vi "MS SQL_Read_TS_Routing.vi"(5 "Pokeyoke?":bool, 6 "PKYK Ref":refnum<vi>[](array[refnum]), 8 "error in (no error)":errorcluster, 11 "Ref in":T2={"MS SQL Connection"=refnum, "UDL File"=path "", "Time"="", "DCODE"="", "WIP+1"=0, "MC No?"=0, "POKAYOKE?"=FALSE, "Expected Result"="", "Result [Status]"="", "Clock"=0.0, "RFID"="", "WIP Queue"=refnum, "TS Parameter"={"ProfitCenterCode"="", "LineCode"="", "WorkOrderNumber"="", "Model"="", "Model_with_Prefix"="", "VendorCode"="", "SetParameterDateCode"="", "PokaYoke"=0, "Target"=1, "Live_DateCode"="", "CustomerPartNumber"="", "Hand"="", "sBarcode"=FALSE, "FCA"=0, "Ent_Stamp"=timestamp(0 s since 1904-01-01), "STS_CD"=0.0}, "Data_Queue"=[], "RFID Serial No."=""} {"TS Parameter"."FCA" format="%01d"; "TS Parameter"."Target" min=1 max=100000; "TS Parameter"."PokaYoke" min=0 max=1}) -> (0 "error out":errorcluster, 1 "Pokeyoke?":bool[](array[boolean]), 2 "Routing?":bool[](array[boolean]), 3 "Ref Out":T2={"MS SQL Connection"=refnum, "UDL File"=path "", "Time"="", "DCODE"="", "WIP+1"=0, "MC No?"=0, "POKAYOKE?"=FALSE, "Expected Result"="", "Result [Status]"="", "Clock"=0.0, "RFID"="", "WIP Queue"=refnum, "TS Parameter"={"ProfitCenterCode"="", "LineCode"="", "WorkOrderNumber"="", "Model"="", "Model_with_Prefix"="", "VendorCode"="", "SetParameterDateCode"="", "PokaYoke"=0, "Target"=1, "Live_DateCode"="", "CustomerPartNumber"="", "Hand"="", "sBarcode"=FALSE, "FCA"=0, "Ent_Stamp"=timestamp(0 s since 1904-01-01), "STS_CD"=0.0}, "Data_Queue"=[], "RFID Serial No."=""} {"TS Parameter"."FCA" format="%01d"; "TS Parameter"."Target" min=1 max=100000; "TS Parameter"."PokaYoke" min=0 max=1})   [LabVIEW 2020]
uses:
  Controls/TD SQL.ctl
  <vilib>/addons/database/Connection.llb/Conn ObjectReference.ctl
  Controls/WIP_State.ctl
  Controls/TS_Parameter.ctl
  <vilib>/Utility/miscctls.llb/LVTextColorsTypeDef.ctl
  MS_Global.vi
  <userlib>/_OpenG.lib/array/array.llb/Search 1D Array (Boolean)__ogtk.vi
  <vilib>/addons/database/NI_Database_API.lvlib
panel:
  in  "TS Parameter":T1={"ProfitCenterCode"="", "LineCode"="", "WorkOrderNumber"="", "Model"="", "Model_with_Prefix"="", "VendorCode"="", "SetParameterDateCode"="", "PokaYoke"=0, "Target"=1, "Live_DateCode"="", "CustomerPartNumber"="", "Hose_Type"="", "Ent_Stamp"=timestamp(0 s since 1904-01-01), "STS_CD"=0.0} {"Target" min=1 max=100000; "PokaYoke" min=0 max=1}
  out "spreadsheet string":string
  out "MachineCode":string[](array[string])
  out "OperationCode":string[](array[string])
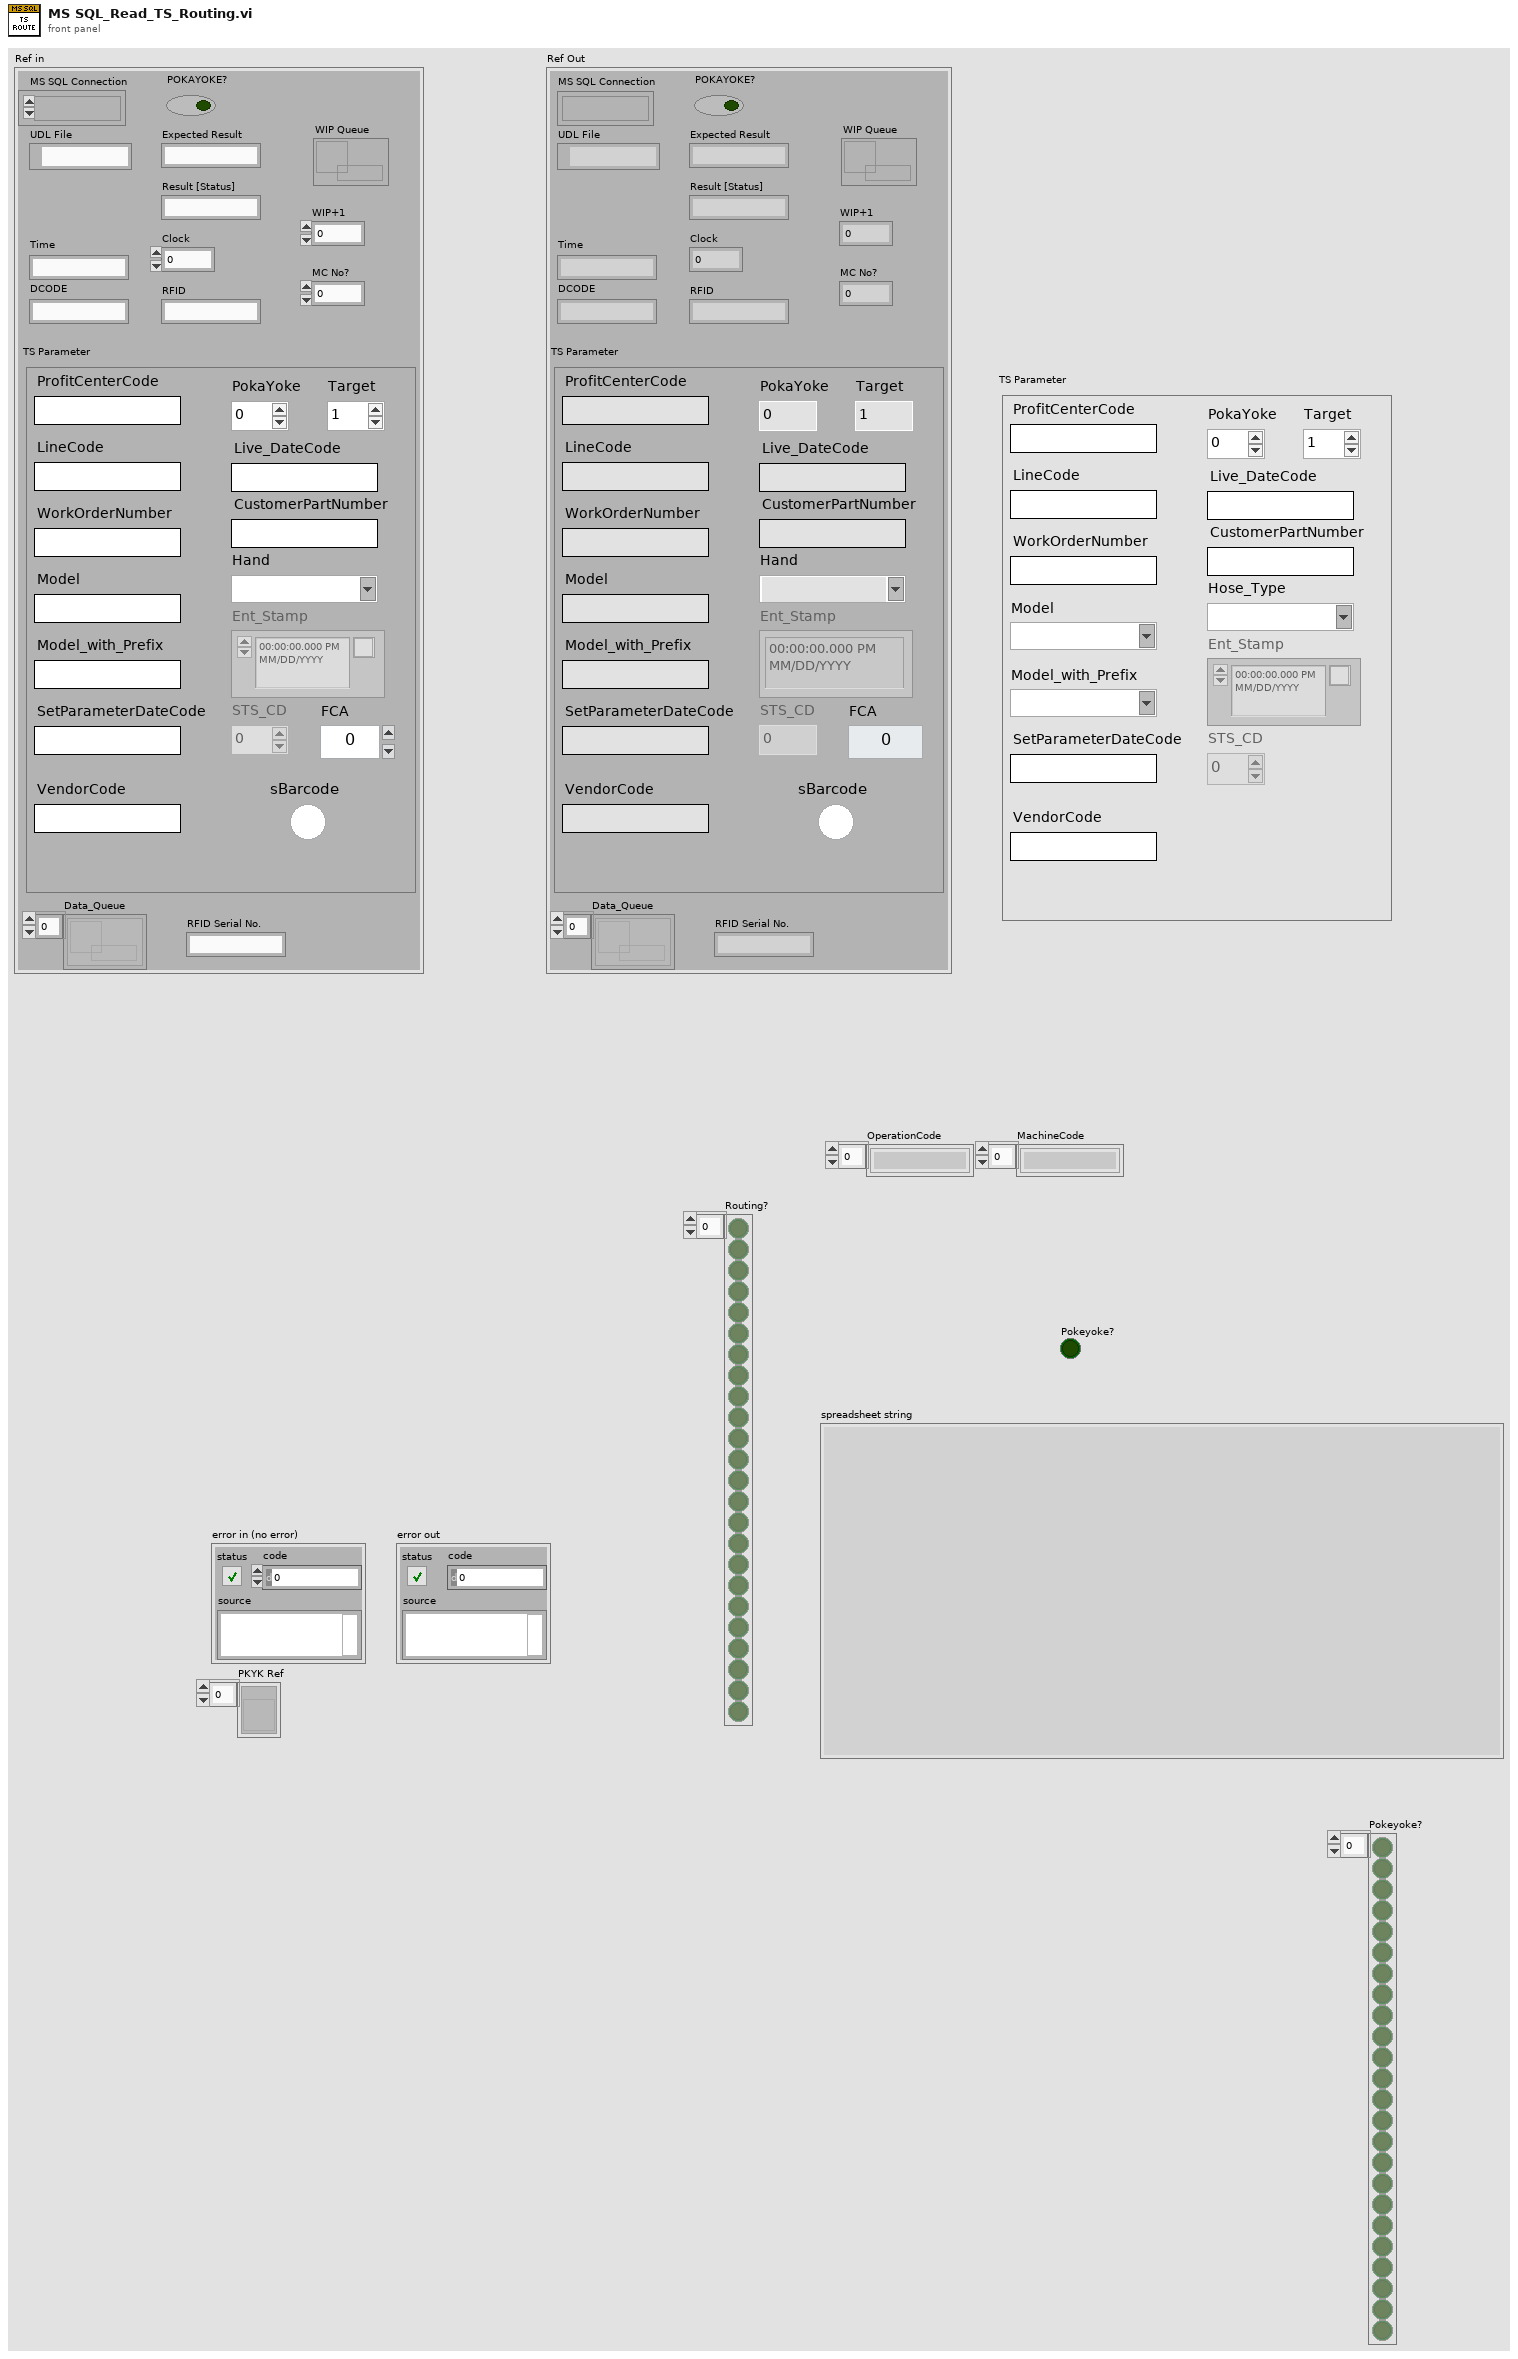
[diagram p1: front panel]
types:
  T1 = cluster{"ProfitCenterCode":string, "LineCode":string, "WorkOrderNumber":string, "Model":string, "Model_with_Prefix":string, "VendorCode":string, "SetParameterDateCode":string, "PokaYoke":i32, "Target":i32, "Live_DateCode":string, "CustomerPartNumber":string, "Hose_Type":string, "Ent_Stamp":timestamp, "STS_CD":dbl}
  T2 = typedef "TD SQL.ctl" = cluster{"MS SQL Connection":T3, "UDL File":path, "Time":string, "DCODE":string, "WIP+1":i64, "MC No?":i32, "POKAYOKE?":bool, "Expected Result":string, "Result [Status]":string, "Clock":dbl, "RFID":string, "WIP Queue":refnum<queue>, "TS Parameter":T4, "Data_Queue":refnum<queue>[], "RFID Serial No.":string}
  T3 = typedef "NI_Database_API.lvlib/Conn ObjectReference.ctl" = refnum<k1>
  T4 = typedef "TS_Parameter.ctl" = cluster{"ProfitCenterCode":string, "LineCode":string, "WorkOrderNumber":string, "Model":string, "Model_with_Prefix":string, "VendorCode":string, "SetParameterDateCode":string, "PokaYoke":i32, "Target":i32, "Live_DateCode":string, "CustomerPartNumber":string, "Hand":string, "sBarcode":bool, "FCA":i32, "Ent_Stamp":timestamp, "STS_CD":dbl}
  T5 = typedef "LVTextColorsTypeDef.ctl" = cluster{"Text Color":u32, "Background Color":u32}
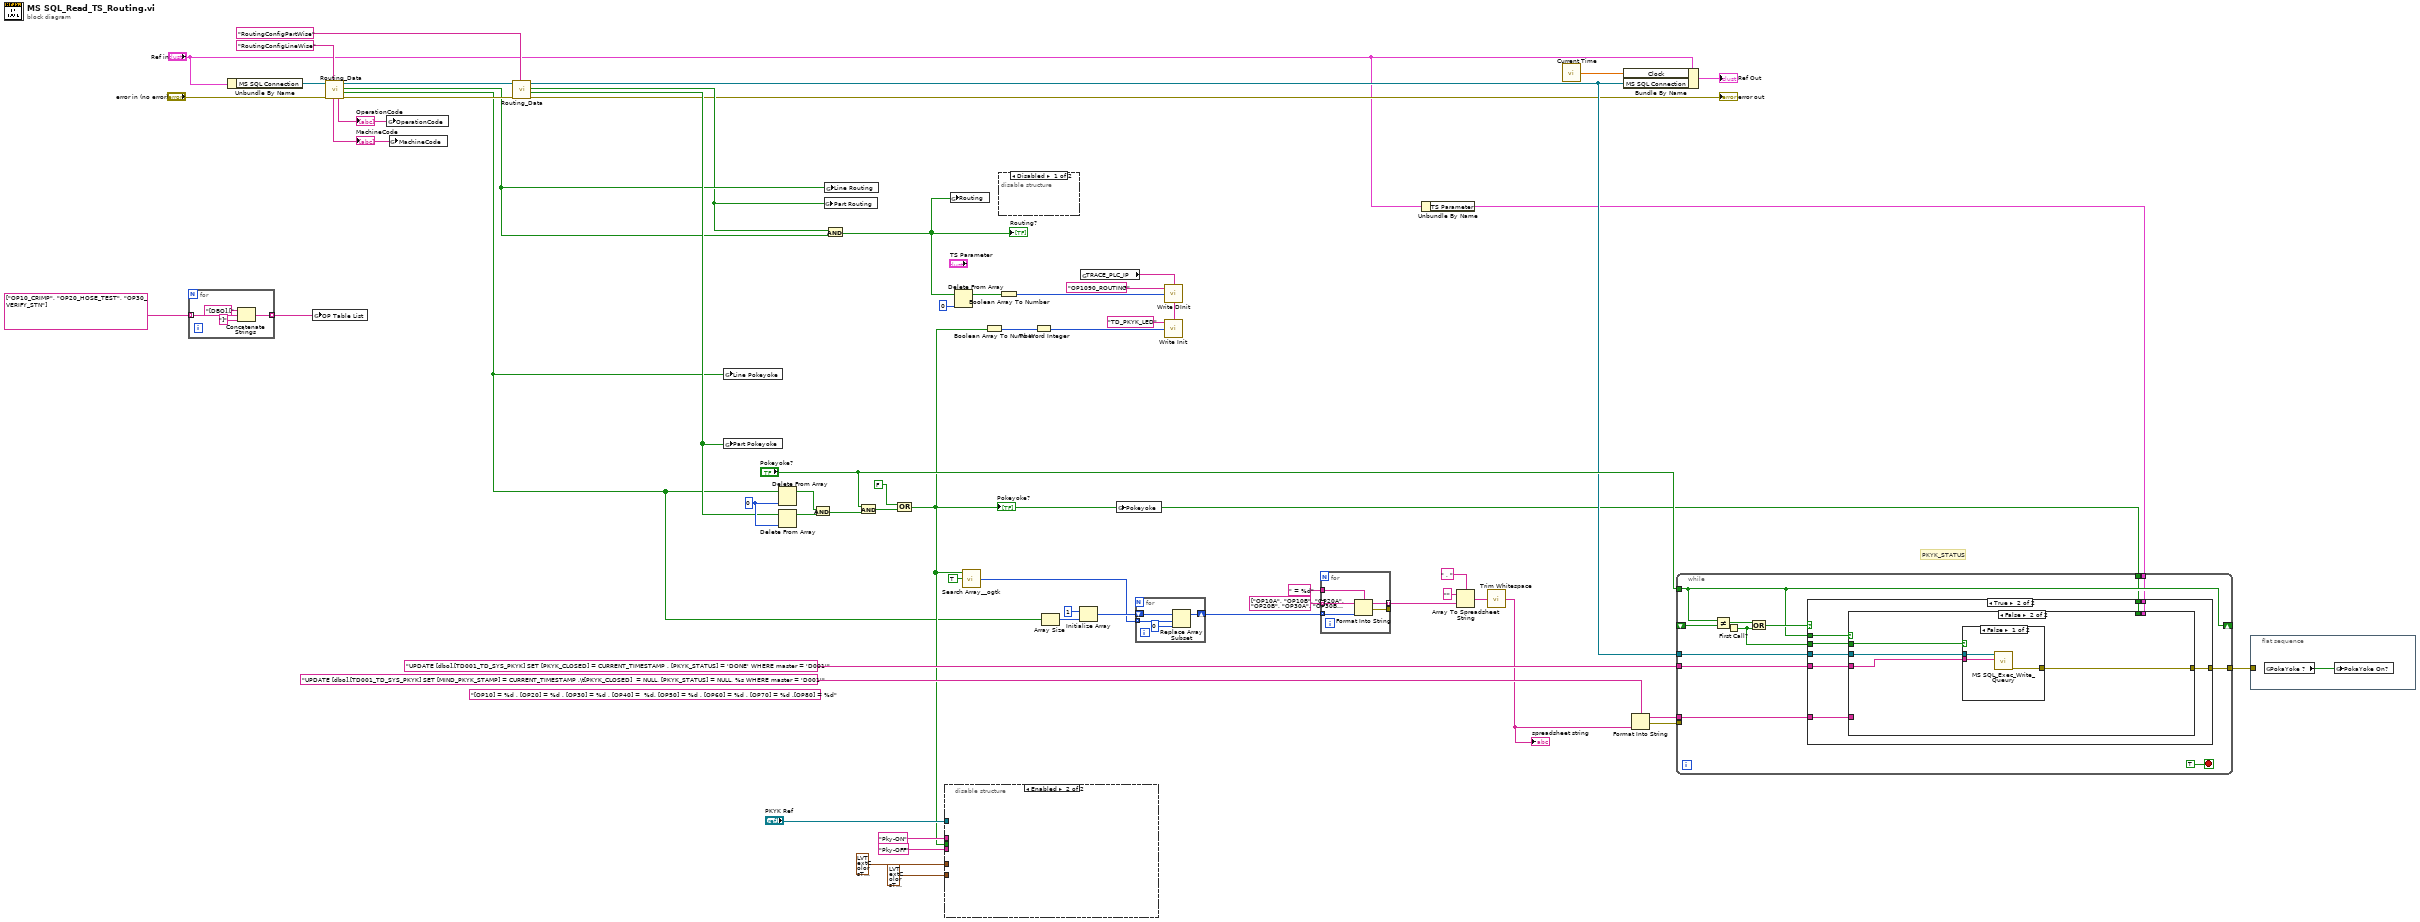
[diagram p0: block diagram]
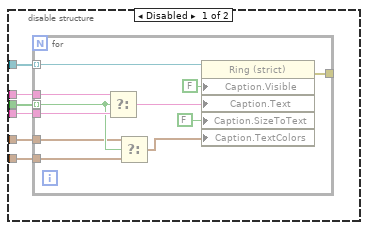
[diagram p3: hidden frame]
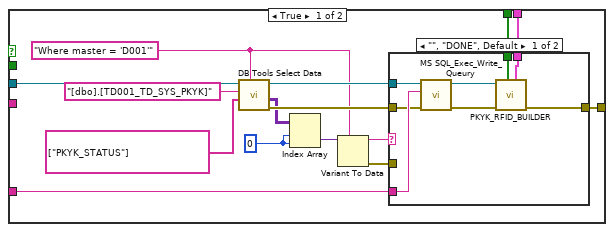
[diagram p5: hidden frame]
diagram:
  (unwired) "[OP10] = %d , [OP20] = %d , [OP30] = %d , [OP40] =  %d, [OP50] = %d , [OP60] = %d , [OP70] = %d ,[OP80] = %d" ("format string")
  w54 = 0 ("index")
  # "PKYK_STATUS"
  n1 = for {
    tunnel: [w62] -> w26 mode=indexing
    tunnel: string[] ["OP10_CRIMP", "OP20_HOSE_TEST", "OP30_VERIFY_STN"] ("tables") -> [w61] mode=indexing
    n2 = Concatenate Strings("[DBO].[" ("string"), w61, "]" ("string")) -> (w62:string)
  }
  n3 = Unbundle By Name("Ref in") -> ("MS SQL Connection"=w59:T3)
  n4 = global write "MS_Global.vi" "OP Table List"(w26) -> ()
  n5 = call "Routing_Data.vi"("Table Name"="RoutingConfigLineWise", "error in (no error)"="error in (no error)", "Refnum in"=w59) -> ("error out"=w35:errorcluster, "Pokeyoke"=w16:bool[], "Routing"=w24:bool[], "Refnum out"=w36:T3, "OperationCode"=w39:string[], "MachineCode"=w38:string[])  [unwired: 3 in]
  "OperationCode" <- w39
  "MachineCode" <- w38
  n6 = global write "MS_Global.vi" "OperationCode"(w39) -> ()
  n7 = global write "MS_Global.vi" "MachineCode"(w38) -> ()
  n8 = call "Routing_Data.vi"("Table Name"="RoutingConfigPartWise", "error in (no error)"=w35, "Refnum in"=w36) -> ("error out"=→"error out":errorcluster, "Pokeyoke"=w33:bool[], "Routing"=w23:bool[], "Refnum out"=w32:T3)  [unwired: 3 in, 2 out]
  n9 = global write "MS_Global.vi" "Line Pokeyoke"(w16) -> ()
  n10 = global write "MS_Global.vi" "Part Pokeyoke"(w33) -> ()
  n11 = Delete From Array(array=w16, index=w54) -> (array with subset deleted=w57:bool[])  [unwired: 1 in, 1 out]
  n12 = Delete From Array(array=w33, index=w54) -> (array with subset deleted=w58:bool[])  [unwired: 1 in, 1 out]
  n13 = And(x=w57, y=w58) -> (x .and. y?=w56:bool[])
  n14 = global write "MS_Global.vi" "Part Routing"(w23) -> ()
  n15 = global write "MS_Global.vi" "Line Routing"(w24) -> ()
  n16 = And(x=w23, y=w24) -> (x .and. y?=w1:bool[])
  "Routing?" <- w1
  n17 = Compound Arithmetic op=AND("Pokeyoke?", w56) -> (w41:bool[])
  n18 = Compound Arithmetic op=OR(FALSE ("Pokeyoke?"), w41) -> (w25:bool[])
  "Pokeyoke?" <- w25
  n19 = disable-structure shown="Enabled" {
    disable-tunnel: "PKYK Ref" -> [w70 _]
    disable-tunnel: "Pky-ON" ("format string") -> [w69 _]
    disable-tunnel: "Pky-OFF" ("format string") -> [w68 _]
    disable-tunnel: T5 {"Text Color"=16777226, "Background Color"=16777216} ("Caption.Text Colors") -> [w67 _]
    disable-tunnel: T5 {"Text Color"=16777226, "Background Color"=46091} ("Caption.Text Colors") -> [w66 _]
    disable-tunnel: w25 -> [w65 _]
    frame Disabled {
      n20 = for {
        tunnel: w70 -> [w81] mode=indexing
        tunnel: w65 -> [w74] mode=indexing
        tunnel: w69 -> [w80]
        tunnel: w68 -> [w79]
        tunnel: [w78] -> _
        tunnel: w67 -> [w73]
        tunnel: w66 -> [w72]
        n21 = Select(t=w80, s=w74, f=w79) -> (s? t:f=w75:string)
        n22 = Select(t=w72, s=w74, f=w73) -> (s? t:f=w71:T5)
        n23 = property class="Ring (strict)"(reference=w81, "Caption.Visible"=FALSE, "Caption.Text"=w75, "Caption.SizeToText"=FALSE ("Caption.Size to Text?"), "Caption.TextColors"=w71) -> (error out=w78:errorcluster)  [unwired: 1 in, 1 out]
      }
    }
    frame Enabled {
    }
  }
  n24 = global write "MS_Global.vi" "Routing"(w1) -> ()
  n25 = Delete From Array(array=w1, index=0) -> (array with subset deleted=w18:bool[])  [unwired: 1 in, 1 out]
  n26 = call-poly <userlib>:"Search Array__ogtk.vi"("Array"=w25, "Element Data"=TRUE) -> ("Indices of Elements"=w50:i32[])  [unwired: 7 in]
  n27 = Boolean Array To Number(Boolean array=w25) -> (number=w44:u32)
  n28 = disable-structure shown="Disabled" {
    frame Disabled {
    }
    frame Enabled {
    }
  }
  n29 = Boolean Array To Number(Boolean array=w18) -> (number=w20:u32)
  n30 = To Word Integer(number=w44) -> (16bit integer=w43:i16)
  n31 = Array Size(array=w16) -> (size(s)=w15:i32)
  n32 = Initialize Array(1 ("index"), w15) -> (w51:i32[])
  n33 = global read "MS_Global.vi" "TRACE_PLC_IP"() -> (w7:string)
  n34 = global write "MS_Global.vi" "Pokeyoke"(w25) -> ()
  n35 = for {
    shift-right: [w84] -> w9
    shift-left: w51 -> [w85]
    tunnel: w50 -> [w82] mode=indexing
    n36 = Replace Array Subset(array=w85, new element=0 ("new element/subarray"), index=w82) -> (w84:i32[])
  }
  n37 = call "Write DInit.vi"("Network Path"=w7, "Int"=w20, "Tag Name"="OP1090_ROUTING" ("Network Path")) -> ()  [unwired: 2 in]
  n38 = call "Write Init.vi"("Network Path"=w7, "Int"=w43, "Tag Name"="TD_PKYK_LED" ("Network Path")) -> ()  [unwired: 1 in, 1 out]
  n39 = for {
    tunnel: string[] ["OP10A", "OP10B", "OP20A", "OP20B", "OP30A", "OP30B", "OP30C", "OP40A", "OP40B", "OP50A", "OP50B", "OP60", "OP70", "OP80"] ("TS_CODE_TAG") -> [w90] mode=indexing
    tunnel: " = %d" ("format string") -> [w89]
    tunnel: [w88] -> w8 mode=indexing
    tunnel: [w87] -> _
    tunnel: w9 -> [w86] mode=indexing
    n40 = Format Into String(format string=w89, initial string=w90, w86) -> (resulting string=w88:string, error out=w87:errorcluster)  [unwired: 1 in]
  }
  n41 = Unbundle By Name("Ref in") -> ("TS Parameter"=w2:T4)
  n42 = Array To Spreadsheet String(delimiter (Tab)=" , ", array=w8, 3:"" ("format string")) -> (spreadsheet string=w12:string)
  n43 = call <vilib>:"Trim Whitespace.vi"("string"=w12) -> ("trimmed string"=w4:string)  [unwired: 1 in]
  "spreadsheet string" <- w4
  n44 = call <userlib>:"Current Time.vi"() -> ("Current Time (Sec)"=w6:dbl)  [unwired: 15 in]
  n45 = Bundle By Name(cluster="Ref in", "Clock"=w6, "MS SQL Connection"=w32) -> (→"Ref Out":T2)
  n46 = Format Into String(format string="UPDATE [dbo].[TD001_TD_SYS_PKYK] SET [MIND_PKYK_STAMP] = CURRENT_TIMESTAMP ,\t[PKYK_CLOSED]  = NULL, [PKYK_STATUS] = NULL, %s WHERE master = 'D001'", w4) -> (resulting string=w47:string, error out=w48:errorcluster)  [unwired: 2 in]
  n47 = while {
    tunnel: "Pokeyoke?" -> [w99]
    shift-right: [w99] -> _
    shift-left: _ -> [w102]
    tunnel: w32 -> [w98]
    tunnel: w48 -> [_]
    tunnel: w47 -> [w97]
    tunnel: "UPDATE [dbo].[TD001_TD_SYS_PKYK] SET [PKYK_CLOSED] = CURRENT_TIMESTAMP , [PKYK_STATUS] = 'DONE' WHERE master = 'D001'" ("format string") -> [w96]
    tunnel: w25 -> [w94]
    tunnel: [w92] -> w5
    tunnel: w2 -> [w91]
    stop <- TRUE stop-if-true
    n48 = Not Equal?(x=w99, y=w102) -> (x != y?=w93:bool)
    n49 = First Call?() -> (First Call?: T/F=w95:bool)
    n50 = Compound Arithmetic op=OR(w93, w95) -> (w100:bool)
    n51 = case shown="True" w100 {
      tunnel: w99 -> [_ w110]
      tunnel: w98 -> [_ w109]
      tunnel: w97 -> [_ w108]
      tunnel: w96 -> [_ w107]
      tunnel: w95 -> [_ w106]
      tunnel: w94 -> [_ w105]
      tunnel: [_ w104] -> w92
      tunnel: w91 -> [_ w103]
      frame False {
      }
      frame True {
        n52 = case shown="False" w110 {
          tunnel: w109 -> [w122 w138]
          tunnel: w108 -> [w125 _]
          tunnel: [w124 w137] -> w104
          tunnel: w107 -> [_ w136]
          tunnel: w106 -> [_ w135]
          tunnel: w105 -> [w112 _]
          tunnel: w103 -> [w111 _]
          frame True {
            w117 = 0 ("index (row)")
            w115 = "Where master = 'D001'" ("condition")
            n53 = call <vilib>:"DB Tools Select Data.vi"("condition"=w115, "columns"=string[] ["PKYK_STATUS"], "table"="[dbo].[TD001_TD_SYS_PKYK]", "connection reference"=w122) -> ("error out"=w120:errorcluster, "data"=w118:variant[][], "connection reference out"=w121:T3)  [unwired: 2 in]
            n54 = Index Array(array=w118, index (row)=w117, index (col)=w117) -> (element=w116:variant)
            n55 = Variant To Data(type=w115, Variant=w116) -> (data=w114:string, error out=w113:errorcluster)  [unwired: 1 in]
            n56 = case shown="\"\", \"DONE\", Default" w114 {
              tunnel: w125 -> [w133 _]
              tunnel: [w128 w134] -> w124
              tunnel: w121 -> [w132 _]
              tunnel: w120 -> [w131 w134]
              tunnel: w113 -> [_ _]
              tunnel: w112 -> [w127 _]
              tunnel: w111 -> [w126 _]
              frame "", "DONE", Default {
                n57 = call "MS SQL_Exec_Write_Queury.vi"("error in (no error)"=w131, "Query"=w133, "Refnum in"=w132) -> ("error out"=w130:errorcluster, "Refnum out"=w129:T3)  [unwired: 7 in]
                n58 = call "PKYK_RFID_BUILDER.vi"("TS Parameter"=w126, "Pokeyoke?"=w127, "error in (no error)"=w130, "MS SQL Connection In"=w129) -> ("error out"=w128:errorcluster)  [unwired: 6 in, 1 out]
              }
              frame "PROCESS" {
              }
            }
          }
          frame False {
            n59 = case shown="False" w135 {
              tunnel: w138 -> [w141 _]
              tunnel: [w140 _] -> w137
              tunnel: w136 -> [w139 _]
              frame False {
                n60 = call "MS SQL_Exec_Write_Queury.vi"("Query"=w139, "Refnum in"=w141) -> ("error out"=w140:errorcluster)  [unwired: 8 in, 1 out]
              }
              frame True {
              }
            }
          }
        }
      }
    }
  }
  n61 = flat-sequence {
    tunnel: w5 -> [_]
    frame #0 {
      n62 = global read "MS_Global.vi" "PokaYoke ?"() -> (w142:bool)
      n63 = global write "MS_Global.vi" "PokaYoke On?"(w142) -> ()
    }
  }
